vi "Send Command.vi"(0 "reference in":refnum<class "CR_master.lvclass">, 5 "message":string, 7 "parameters":string, 9 "data":variant, 11 "error in (no error)":errorcluster, 12 "response?":bool, 13 "timeout":i32) -> (4 "reference out":refnum<class "CR_master.lvclass">, 6 "status":string, 8 "reponse":string, 10 "data":variant, 15 "error out":errorcluster)   [LabVIEW 2019, in "CommandResponse communication.lvlib" / "CR_master.lvclass"]
doc: "Sends command as message + variant data and optionally awaits for response message and error"
uses:
  CR_master.lvclass
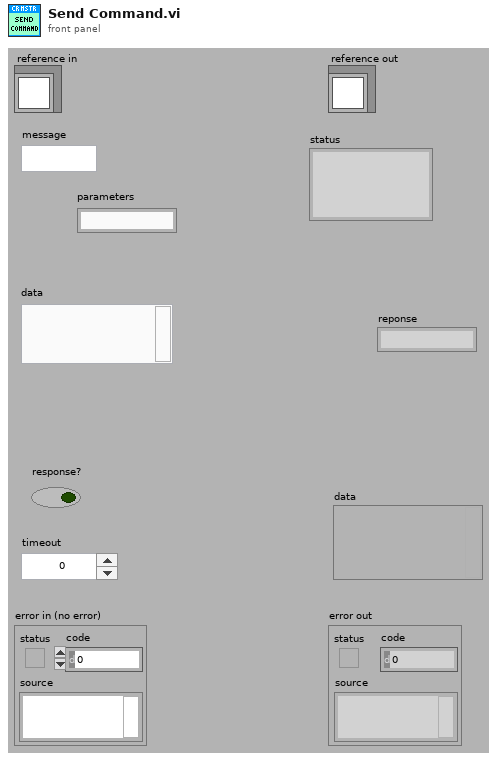
[diagram p1: front panel]
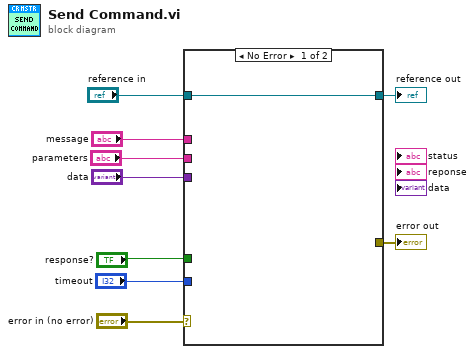
[diagram p0: block diagram]
diagram:
  n1 = case shown="No Error" "error in (no error)" {
    selector: "error in (no error)" -> [_ w12]
    tunnel: [_ w12] -> w8
    tunnel: [w10 w11] -> w6
    tunnel: "reference in" -> [w10 w11]
    tunnel: "message" -> [_ _]
    tunnel: "parameters" -> [_ _]
    tunnel: "response?" -> [_ _]
    tunnel: "timeout" -> [_ _]
    tunnel: "data" -> [_ _]
    frame No Error {
    }
    frame Error {
    }
  }
  "error out" <- w8
  "reference out" <- w6
